vi "Create GUID Substitution Map.vi"(11 "guids":set{string}(c389)) -> (3 "guid map":map{string, string}(c390))   [LabVIEW 2020, in "GUID Tool.lvlib"]
uses:
  GUID Tool.lvlib
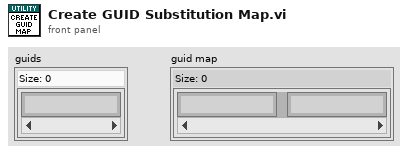
[diagram p1: front panel]
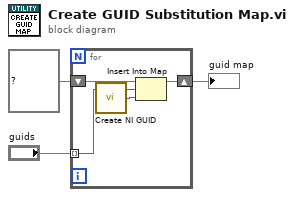
[diagram p0: block diagram]
diagram:
  n1 = for {
    tunnel: "guids" -> [w6] mode=indexing
    shift-right: [w4] -> w1
    shift-left: map{string, string} {} ("map in") -> [w5]
    n2 = call <vilib>:"Create NI GUID.vi"() -> ("NI GUID"=w7:string)
    n3 = Insert Into Map(map in=w5, key=w6, value=w7) -> (map out=w4:map{string, string})  [unwired: 2 out]
  }
  "guid map" <- w1
